vi "StoreDefaultParams.vi"(8 "error in (no error)":errorcluster, 10 "DefaultINIParams":T1={"Handle"="", "eFunction"=0, "dRange"=0.0, "dResolution"=0.0, "eTriggerSource"=0, "dTriggerDelay"=0.0, "iMaxTimeMilliseconds"=0, "eMeasCompleteDest"=0, "iTriggerCount"=0, "iSampleCount"=0, "eSampleClock"=0, "dSampleInterval"=0.0, "iMaxTimeMillisecondsMultiPoint"=0, "iArraySize"=0, "dMinFreq"=0.0, "dMaxFreq"=0.0, "dFrequencyVoltageRange"=0.0, "eEdge"=10280, "sSource"="", "eEdgeSample"=10280, "sSourceSample"="", "eSampleMode"=10178} {"eSampleMode" items=["Finite Samples"=10178, "Continuous Samples"=10123, "Hardware Timed Single Point"=12522]; "eEdgeSample" items=["Rising"=10280, "Falling"=10171]; "eEdge" items=["Rising"=10280, "Falling"=10171]; "eSampleClock" items=["NULL"=0, "Immediate"=1, "External"=2, "Software Trigger"=3, "Interval"=10]; "eMeasCompleteDest" items=["None"=0, "External"=2]; "eTriggerSource" items=["NULL", "Immediate", "External", "Software Trigger"]; "eFunction" items=["NULL"=0, "DC Volts"=1, "AC Volts"=2, "DC Current"=3, "AC Current"=4, "Frequency"=104, "AC Coupled Direct Sampling"=1005]}, 11 "NISTNiPxi6123 in":refnum<class "NiPxi6123.lvclass">) -> (0 "error out":errorcluster, 3 "NISTNiPxi6123 out":refnum<class "NiPxi6123.lvclass">)   [LabVIEW 2014]
uses:
  NiPxi6123.lvclass
  NISTSamplerPluginsBaseClass/TypeDefs/DefaultINIParams.ctl
  NISTSamplerPluginsBaseClass/SamplerPluginsBase.lvclass
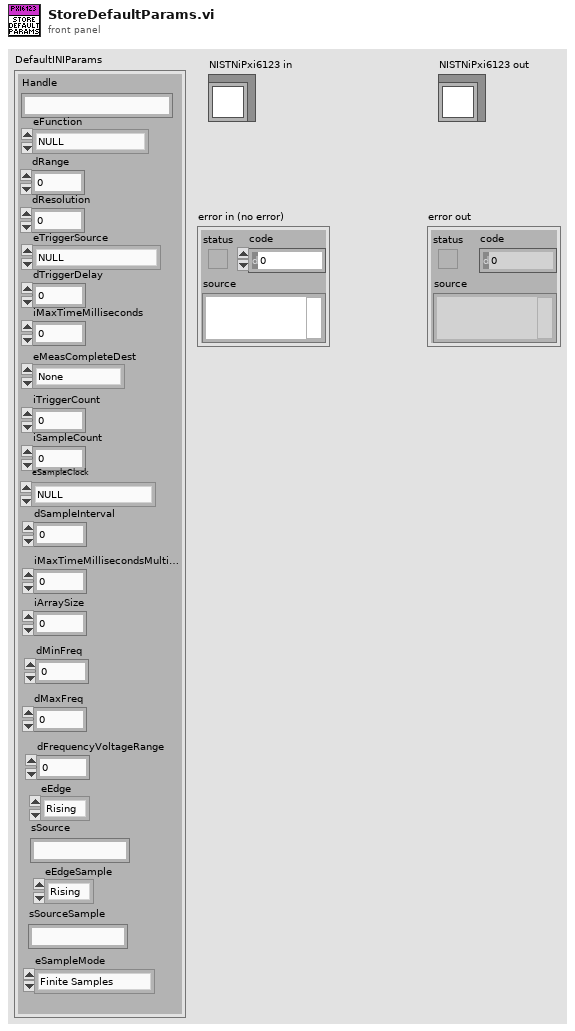
[diagram p1: front panel]
types:
  T1 = typedef "SamplerPlugins.lvlib/SamplerPluginsBase.lvclass/DefaultINIParams.ctl" = cluster{"Handle":string, "eFunction":u16, "dRange":dbl, "dResolution":dbl, "eTriggerSource":u16, "dTriggerDelay":dbl, "iMaxTimeMilliseconds":i32, "eMeasCompleteDest":u16, "iTriggerCount":i32, "iSampleCount":i32, "eSampleClock":u16, "dSampleInterval":dbl, "iMaxTimeMillisecondsMultiPoint":i32, "iArraySize":i32, "dMinFreq":dbl, "dMaxFreq":dbl, "dFrequencyVoltageRange":dbl, "eEdge":u16, "sSource":string, "eEdgeSample":u16, "sSourceSample":string, "eSampleMode":i32}
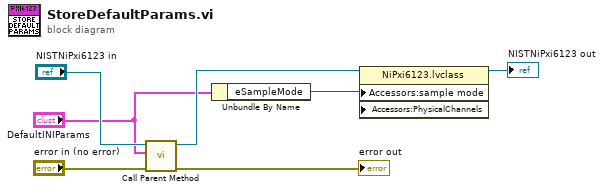
[diagram p0: block diagram]
diagram:
  n1 = call-parent "Call Parent Method"("error in (no error)"="error in (no error)", "DefaultINIParams"="DefaultINIParams", "NISTSamplerPluginsBase in"="NISTNiPxi6123 in") -> ("error out"=→"error out":errorcluster, "NISTSamplerPluginsBase out"=w6:refnum<class "NiPxi6123.lvclass">)  [unwired: 7 in]
  n2 = Unbundle By Name("DefaultINIParams") -> ("eSampleMode"=w1:i32)
  n3 = property class="NiPxi6123.lvclass" props=["Accessors:sample mode", "Accessors:PhysicalChannels"](reference=w6, "Accessors:sample mode"=w1) -> (reference out=→"NISTNiPxi6123 out":refnum<class "NiPxi6123.lvclass">)  [unwired: 2 in, 1 out]
